vi "rsidr_core_global.vi"() -> ()   [LabVIEW 2020, in "Rohde&Schwarz RTx Oscilloscopes.lvlib"] (continued)
Table"="", "Read Callback"="", "Write Callback"="", "Supported Models"="", "Instrument Options"="K15", "Flags"=0, "Help"="Displays or hides the segment table on the screen.\n\nAvailable Repeated Capabilities:\nMath: MA1, MA2, MA3, MA4, MA5\r\n\nRemote-control command(s):\nCALCulate:MATH<m>:HISTory:TTABle[:ENABle]"}, {"Level"=4, "Class Only"=FALSE, "Identifier"="RSRTX_ATTR_HISTORY_MATH_EXPORT_NAME", "Descriptive Name"="History Math Export Name", "Data Type"=2, "Command"="CALC:MATH{Math}:HIST:EXP:NAME", "Access"=2, "Range Table"="", "Read Callback"="", "Write Callback"="", "Supported Models"="RTM|RTA", "Instrument Options"="", "Flags"=0, "Help"="History export file name.\n\nAvailable Repeated Capabilities:\nMath: MA1, MA2, MA3, MA4, MA5\r\n\nRemote-control command(s):\nCALCulate:MATH<m>:HISTory:EXPort:NAME"}, {"Level"=4, "Class Only"=FALSE, "Identifier"="RSRTX_ATTR_HISTORY_MATH_EXPORT_SAVE", "Descriptive Name"="History Math Export Save", "Data Type"=4, "Command"="CALC:MATH{Math}:HIST:EXP:SAVE", "Access"=1, "Range Table"="", "Read Callback"="", "Write Callback"="", "Supported Models"="RTM|RTA", "Instrument Options"="", "Flags"=0, "Help"="Exports history.\n\nAvailable Repeated Capabilities:\nMath: MA1, MA2, MA3, MA4, MA5\r\n\nRemote-control command(s):\nCALCulate:MATH<m>:HISTory:EXPort:SAVE"}, {"Level"=3, "Class Only"=TRUE, "Identifier"="", "Descriptive Name"="Protocol", "Data Type"=0, "Command"="", "Access"=0, "Range Table"="", "Read Callback"="", "Write Callback"="", "Supported Models"="", "Instrument Options"="", "Flags"=0, "Help"="Configures history for protocol."}, {"Level"=4, "Class Only"=FALSE, "Identifier"="RSRTX_ATTR_HISTORY_PROTOCOL_CURRENT_ACQUISITION", "Descriptive Name"="History Protocol Current Acquisition", "Data Type"=0, "Command"="BUS{SerialBus}:HIST:CURR", "Access"=2, "Range Table"="", "Read Callback"="", "Write Callback"="", "Supported Models"="", "Instrument Options"="K15", "Flags"=0, "Help"="Accesses a particular acquisition segment in the memory to display it. The query returns the index of the segment that is shown.\nThere are two ways to enter the index.\nNegative index count: the newest segment has the index 0, older segments have a negative index: -(n-1), .... -1 , 0\nPositive index count: the oldest segment has the index 1, and the newest segment has the index n: 1, 2,..., n\nwhere n is the number of acquired segments.\n\nAvailable Repeated Capabilities:\nSerialBus: SB1, SB2, SB3, SB4\r\n\nRemote-control command(s):\nBUS<b>:HISTory:CURRent"}, {"Level"=4, "Class Only"=FALSE, "Identifier"="RSRTX_ATTR_HISTORY_PROTOCOL_PLAYER", "Descriptive Name"="History Protocol Player", "Data Type"=0, "Command"="BUS{SerialBus}:HIST:PLAY:STAT", "Access"=2, "Range Table"="rsrtx_rngHistoryPlayer", "Read Callback"="", "Write Callback"="", "Supported Models"="", "Instrument Options"="K15", "Flags"=0, "Help"="Starts and stops the replay of the history segments.\n\nAvailable Repeated Capabilities:\nSerialBus: SB1, SB2, SB3, SB4\r\n\nRemote-control command(s):\nBUS<b>:HISTory:PLAYer:STATe"}, {"Level"=4, "Class Only"=FALSE, "Identifier"="RSRTX_ATTR_HISTORY_PROTOCOL_START_ACQUISITION", "Descriptive Name"="History Protocol Start Acquisition", "Data Type"=0, "Command"="BUS{SerialBus}:HIST:STAR", "Access"=2, "Range Table"="", "Read Callback"="", "Write Callback"="", "Supported Models"="", "Instrument Options"="K15", "Flags"=0, "Help"="Sets the index of the oldest segment to be displayed.\nThere are two ways to enter the index.\nNegative index count: the newest segment has the index 0, older segments have a negative index: -(n-1), .... -1 , 0\nPositive index count: the oldest segment has the index 1, and the newest segment has the index n: 1, 2,..., n\nwhere n is the number of acquired segments.\n\nAvailable Repeated Capabilities:\nSerialBus: SB1, SB2, SB3, SB4\r\n\nRemote-control command(s):\nBUS<b>:HISTory:STARt"}, {"Level"=4, "Class Only"=FALSE, "Identifier"="RSRTX_ATTR_HISTORY_PROTOCOL_STOP_ACQUISITION", "Descriptive Name"="History Protocol Stop Acquisition", "Data Type"=0, "Command"="BUS{SerialBus}:HIST:STOP", "Access"=2, "Range Table"="", "Read Callback"="", "Write Callback"="", "Supported Models"="", "Instrument Options"="K15", "Flags"=0, "Help"="Sets the index of the latest segment to be displayed.\nThere are two ways to enter the index.\nNegative index count: the newest segment has the index 0, older segments have a negative index: -(n-1), .... -1 , 0\nPositive index count: the oldest segment has the index 1, and the newest segment has the index n: 1, 2,..., n\nwhere n is the number of acquired segments.\n\nAvailable Repeated Capabilities:\nSerialBus: SB1, SB2, SB3, SB4\r\n\nRemote-control command(s):\nBUS<b>:HISTory:STOP"}, {"Level"=4, "Class Only"=FALSE, "Identifier"="RSRTX_ATTR_HISTORY_PROTOCOL_PLAY_ALL", "Descriptive Name"="History Protocol Play All", "Data Type"=3, "Command"="BUS{SerialBus}:HIST:PALL", "Access"=2, "Range Table"="", "Read Callback"="", "Write Callback"="", "Supported Models"="", "Instrument Options"="K15", "Flags"=0, "Help"="Enables the replay of all acquired segments.\n\nAvailable Repeated Capabilities:\nSerialBus: SB1, SB2, SB3, SB4\r\n\nRemote-control command(s):\nBUS<b>:HISTory:PALL"}, {"Level"=4, "Class Only"=FALSE, "Identifier"="RSRTX_ATTR_HISTORY_PROTOCOL_SPEED", "Descriptive Name"="History Protocol Speed", "Data Type"=0, "Command"="BUS{SerialBus}:HIST:PLAY:SPE", "Access"=2, "Range Table"="rsrtx_rngHistorySpeed", "Read Callback"="", "Write Callback"="", "Supported Models"="", "Instrument Options"="K15", "Flags"=0, "Help"="Sets the speed of the history replay.\n\nAvailable Repeated Capabilities:\nSerialBus: SB1, SB2, SB3, SB4\r\n\nRemote-control command(s):\nBUS<b>:HISTory:PLAYer:SPEed"}, {"Level"=4, "Class Only"=FALSE, "Identifier"="RSRTX_ATTR_HISTORY_PROTOCOL_REPEAT", "Descriptive Name"="History Protocol Repeat", "Data Type"=3, "Command"="BUS{SerialBus}:HIST:REPL", "Access"=2, "Range Table"="", "Read Callback"="", "Write Callback"="", "Supported Models"="", "Instrument Options"="K15", "Flags"=0, "Help"="If set to true, the replay of the selected history segments repeats automatically.\n\nAvailable Repeated Capabilities:\nSerialBus: SB1, SB2, SB3, SB4\r\n\nRemote-control command(s):\nBUS<b>:HISTory:REPLay"}, {"Level"=4, "Class Only"=FALSE, "Identifier"="RSRTX_ATTR_HISTORY_PROTOCOL_ACQUISITON_RELATIVE_TIME", "Descriptive Name"="History Protocol Acquisiton Relative Time", "Data Type"=1, "Command"="BUS{SerialBus}:HIST:TSR?", "Access"=0, "Range Table"="", "Read Callback"="", "Write Callback"="", "Supported Models"="", "Instrument Options"="K15", "Flags"=0, "Help"="Returns the time difference of the selected segment to the newest segment.\n\nAvailable Repeated Capabilities:\nSerialBus: SB1, SB2, SB3, SB4\r\n\nRemote-control command(s):\nBUS<b>:HISTory:TSRelative?"}, {"Level"=4, "Class Only"=FALSE, "Identifier"="RSRTX_ATTR_HISTORY_PROTOCOL_ALL_DATES", "Descriptive Name"="History Protocol All Dates", "Data Type"=2, "Command"="BUS{SerialBus}:HIST:TSD:ALL?", "Access"=0, "Range Table"="", "Read Callback"="", "Write Callback"="", "Supported Models"="", "Instrument Options"="", "Flags"=0, "Help"="Returns the dates of all history segments.\n\nAvailable Repeated Capabilities:\nSerialBus: SB1, SB2, SB3, SB4\r\n\nRemote-control command(s):\nBUS<b>:HISTory:TSDate:ALL?"}, {"Level"=4, "Class Only"=FALSE, "Identifier"="RSRTX_ATTR_HISTORY_PROTOCOL_ALL_TIME_DIFFERENCES", "Descriptive Name"="History Protocol All Time Differences", "Data Type"=2, "Command"="BUS{SerialBus}:HIST:TSR:ALL?", "Access"=0, "Range Table"="", "Read Callback"="", "Write Callback"="", "Supported Models"="", "Instrument Options"="", "Flags"=0, "Help"="Returns the time differences to the newest acquisition of all history segments.\n\nAvailable Repeated Capabilities:\nSerialBus: SB1, SB2, SB3, SB4\r\n\nRemote-control command(s):\nBUS<b>:HISTory:TSRelative:ALL?"}, {"Level"=4, "Class Only"=FALSE, "Identifier"="RSRTX_ATTR_HISTORY_PROTOCOL_ALL_DAYTIMES", "Descriptive Name"="History Protocol All Daytimes", "Data Type"=2, "Command"="BUS{SerialBus}:HIST:TSAB:ALL?", "Access"=0, "Range Table"="", "Read Callback"="", "Write Callback"="", "Supported Models"="", "Instrument Options"="", "Flags"=0, "Help"="Returns the absolute daytimes of all history segments.\n\nAvailable Repeated Capabilities:\nSerialBus: SB1, SB2, SB3, SB4\r\n\nRemote-control command(s):\nBUS<b>:HISTory:TSABsolute:ALL?"}, {"Level"=4, "Class Only"=FALSE, "Identifier"="RSRTX_ATTR_HISTORY_PROTOCOL_PLAYER_CONTROL_ENABLE", "Descriptive Name"="History Protocol Player Control Enable", "Data Type"=3, "Command"="BUS{SerialBus}:HIST:CONT", "Access"=2, "Range Table"="", "Read Callback"="", "Write Callback"="", "Supported Models"="", "Instrument Options"="K15", "Flags"=0, "Help"="Displays or hides the history player on the screen.\n\nAvailable Repeated Capabilities:\nSerialBus: SB1, SB2, SB3, SB4\r\n\nRemote-control command(s):\nBUS<b>:HISTory:CONTrol[:ENABle]"}, {"Level"=4, "Class Only"=FALSE, "Identifier"="RSRTX_ATTR_HISTORY_PROTOCOL_TIME_TABLE_ENABLE", "Descriptive Name"="History Protocol Time Table Enable", "Data Type"=3, "Command"="BUS{SerialBus}:HIST:TTAB", "Access"=2, "Range Table"="", "Read Callback"="", "Write Callback"="", "Supported Models"="", "Instrument Options"="K15", "Flags"=0, "Help"="Displays or hides the segment table on the screen.\n\nAvailable Repeated Capabilities:\nSerialBus: SB1, SB2, SB3, SB4\r\n\nRemote-control command(s):\nBUS<b>:HISTory:TTABle[:ENABle]"}, {"Level"=4, "Class Only"=FALSE, "Identifier"="RSRTX_ATTR_HISTORY_PROTOCOL_EXPORT_NAME", "Descriptive Name"="History Protocol Export Name", "Data Type"=2, "Command"="BUS{SerialBus}:HIST:EXP:NAME", "Access"=2, "Range Table"="", "Read Callback"="", "Write Callback"="", "Supported Models"="", "Instrument Options"="", "Flags"=0, "Help"="History export file name.\n\nAvailable Repeated Capabilities:\nSerialBus: SB1, SB2, SB3, SB4\r\n\nRemote-control command(s):\nBUS<b>:HISTory:EXPort:NAME"}, {"Level"=4, "Class Only"=FALSE, "Identifier"="RSRTX_ATTR_HISTORY_PROTOCOL_EXPORT_SAVE", "Descriptive Name"="History Protocol Export Save", "Data Type"=4, "Command"="BUS{SerialBus}:HIST:EXP:SAVE", "Access"=1, "Range Table"="", "Read Callback"="", "Write Callback"="", "Supported Models"="", "Instrument Options"="", "Flags"=0, "Help"="Exports history.\n\nAvailable Repeated Capabilities:\nSerialBus: SB1, SB2, SB3, SB4\r\n\nRemote-control command(s):\nBUS<b>:HISTory:EXPort:SAVE"}, {"Level"=3, "Class Only"=TRUE, "Identifier"="", "Descriptive Name"="Spectrum", "Data Type"=0, "Command"="", "Access"=0, "Range Table"="", "Read Callback"="", "Write Callback"="", "Supported Models"="", "Instrument Options"="", "Flags"=0, "Help"="Contains attributes for Spectrum History."}, {"Level"=4, "Class Only"=FALSE, "Identifier"="RSRTX_ATTR_HISTORY_SPECTRUM_CURRENT_ACQUISITION", "Descriptive Name"="History Spectrum Current Acquisition", "Data Type"=0, "Command"="SPEC:HIST:CURR", "Access"=2, "Range Table"="", "Read Callback"="", "Write Callback"="", "Supported Models"="", "Instrument Options"="K15", "Flags"=0, "Help"="Accesses a particular acquisition segment in the memory to display it. The query returns the index of the segment that is shown.\n\nAvailable Repeated Capabilities:\nNone\n\nRemote-control command(s):\nSPECtrum:HISTory:CURRent"}, {"Level"=4, "Class Only"=FALSE, "Identifier"="RSRTX_ATTR_HISTORY_SPECTRUM_PLAYER", "Descriptive Name"="History Spectrum Player", "Data Type"=0, "Command"="SPEC:HIST:PLAY:STAT", "Access"=2, "Range Table"="rsrtx_rngHistoryPlayer", "Read Callback"="", "Write Callback"="", "Supported Models"="", "Instrument Options"="K15", "Flags"=0, "Help"="Starts and stops the replay of the history segments.\n\nAvailable Repeated Capabilities:\nNone\n\nRemote-control command(s):\nSPECtrum:HISTory:PLAYer:STATe"}, {"Level"=4, "Class Only"=FALSE, "Identifier"="RSRTX_ATTR_HISTORY_SPECTRUM_START_ACQUISITION", "Descriptive Name"="History Spectrum Start Acquisition", "Data Type"=0, "Command"="SPEC:HIST:STAR", "Access"=2, "Range Table"="", "Read Callback"="", "Write Callback"="", "Supported Models"="", "Instrument Options"="K15", "Flags"=0, "Help"="Sets the index of the oldest segment to be displayed.\nThere are two ways to enter the index.\nNegative index count: the newest segment has the index 0, older segments have a negative index: -(n-1), .... -1 , 0\nPositive index count: the oldest segment has the index 1, and the newest segment has the index n: 1, 2,..., n\nwhere n is the number of acquired segments.\n\nAvailable Repeated Capabilities:\nNone\n\nRemote-control command(s):\nSPECtrum:HISTory:STARt"}, {"Level"=4, "Class Only"=FALSE, "Identifier"="RSRTX_ATTR_HISTORY_SPECTRUM_STOP_ACQUISITION", "Descriptive Name"="History Spectrum Stop Acquisition", "Data Type"=0, "Command"="SPEC:HIST:STOP", "Access"=2, "Range Table"="", "Read Callback"="", "Write Callback"="", "Supported Models"="", "Instrument Options"="K15", "Flags"=0, "Help"="Sets the index of the latest segment to be displayed.\nThere are two ways to enter the index.\nNegative index count: the newest segment has the index 0, older segments have a negative index: -(n-1), .... -1 , 0\nPositive index count: the oldest segment has the index 1, and the newest segment has the index n: 1, 2,..., n\nwhere n is the number of acquired segments.\n\nAvailable Repeated Capabilities:\nNone\n\nRemote-control command(s):\nSPECtrum:HISTory:STOP"}, {"Level"=4, "Class Only"=FALSE, "Identifier"="RSRTX_ATTR_HISTORY_SPECTRUM_PLAY_ALL", "Descriptive Name"="History Spectrum Play All", "Data Type"=3, "Command"="SPEC:HIST:PALL", "Access"=2, "Range Table"="", "Read Callback"="", "Write Callback"="", "Supported Models"="", "Instrument Options"="K15", "Flags"=0, "Help"="Enables the replay of all acquired segments.\n\nAvailable Repeated Capabilities:\nNone\n\nRemote-control command(s):\nSPECtrum:HISTory:PALL"}, {"Level"=4, "Class Only"=FALSE, "Identifier"="RSRTX_ATTR_HISTORY_SPECTRUM_SPEED", "Descriptive Name"="History Spectrum Speed", "Data Type"=0, "Command"="SPEC:HIST:PLAY:SPE", "Access"=2, "Range Table"="rsrtx_rngHistorySpeed", "Read Callback"="", "Write Callback"="", "Supported Models"="", "Instrument Options"="K15", "Flags"=0, "Help"="Sets the speed of the history replay.\n\nAvailable Repeated Capabilities:\nNone\n\nRemote-control command(s):\nSPECtrum:HISTory:PLAYer:SPEed"}, {"Level"=4, "Class Only"=FALSE, "Identifier"="RSRTX_ATTR_HISTORY_SPECTRUM_REPEAT", "Descriptive Name"="History Spectrum Repeat", "Data Type"=3, "Command"="SPEC:HIST:REPL", "Access"=2, "Range Table"="", "Read Callback"="", "Write Callback"="", "Supported Models"="", "Instrument Options"="K15", "Flags"=0, "Help"="If set to true, the replay of the selected history segments repeats automatically.\n\nAvailable Repeated Capabilities:\nNone\n\nRemote-control command(s):\nSPECtrum:HISTory:REPLay"}, {"Level"=4, "Class Only"=FALSE, "Identifier"="RSRTX_ATTR_HISTORY_SPECTRUM_ACQUISITION_RELATIVE_TIME", "Descriptive Name"="History Spectrum Acquisition Relative Time", "Data Type"=1, "Command"="SPEC:HIST:TSR?", "Access"=0, "Range Table"="", "Read Callback"="", "Write Callback"="", "Supported Models"="", "Instrument Options"="", "Flags"=0, "Help"="Returns the time difference of the selected segment to the newest segment. To select a segment, use RSRTX_ATTR_HISTORY_CHANNEL_CURRENT_ACQUISITION. The newest segment has index 0.\n\nAvailable Repeated Capabilities:\nNone\n\nRemote-control command(s):\nSPECtrum:HISTory:TSRelative?"}, {"Level"=4, "Class Only"=FALSE, "Identifier"="RSRTX_ATTR_HISTORY_SPECTRUM_ALL_DATES", "Descriptive Name"="History Spectrum All Dates", "Data Type"=2, "Command"="SPEC:HIST:TSD:ALL?", "Access"=0, "Range Table"="", "Read Callback"="", "Write Callback"="", "Supported Models"="", "Instrument Options"="", "Flags"=0, "Help"="Returns the dates of all history segments as a list of comma-separated list of year, month, and day values. The list starts with the oldest segment, and the newest segment is the last one.\n\nAvailable Repeated Capabilities:\nNone\n\nRemote-control command(s):\nSPECtrum:HISTory:TSDate:ALL?"}, {"Level"=4, "Class Only"=FALSE, "Identifier"="RSRTX_ATTR_HISTORY_SPECTRUM_ALL_TIME_DIFFERENCES", "Descriptive Name"="History Spectrum All Time Differences", "Data Type"=2, "Command"="SPEC:HIST:TSR:ALL?", "Access"=0, "Range Table"="", "Read Callback"="", "Write Callback"="", "Supported Models"="", "Instrument Options"="", "Flags"=0, "Help"="Returns the time differences to the newest acquisition of all history segments.\n\nAvailable Repeated Capabilities:\nNone\n\nRemote-control command(s):\nSPECtrum:HISTory:TSRelative:ALL?"}, {"Level"=4, "Class Only"=FALSE, "Identifier"="RSRTX_ATTR_HISTORY_SPECTRUM_ALL_DAYTIMES", "Descriptive Name"="History Spectrum All Daytimes", "Data Type"=2, "Command"="SPEC:HIST:TSAB:ALL?", "Access"=0, "Range Table"="", "Read Callback"="", "Write Callback"="", "Supported Models"="", "Instrument Options"="", "Flags"=0, "Help"="Returns the absolute daytimes of all history segments.\n\nAvailable Repeated Capabilities:\nNone\n\nRemote-control command(s):\nSPECtrum:HISTory:TSABsolute:ALL?"}, {"Level"=4, "Class Only"=FALSE, "Identifier"="RSRTX_ATTR_HISTORY_SPECTRUM_EXPORT_NAME", "Descriptive Name"="History Spectrum Export Name", "Data Type"=2, "Command"="SPEC:HIST:EXP:NAME", "Access"=2, "Range Table"="", "Read Callback"="", "Write Callback"="", "Supported Models"="", "Instrument Options"="K15", "Flags"=0, "Help"="Defines the path and filename of the spectrum analysis timestamps file. The file format is CSV. If the file already exists, it will be overwritten.\n\nAvailable Repeated Capabilities:\nNone\n\nRemote-control command(s):\nSPECtrum:HISTory:EXPort:NAME"}, {"Level"=4, "Class Only"=FALSE, "Identifier"="RSRTX_ATTR_HISTORY_SPECTRUM_EXPORT_SAVE", "Descriptive Name"="History Spectrum Export Save", "Data Type"=4, "Command"="SPEC:HIST:EXP:SAVE", "Access"=1, "Range Table"="", "Read Callback"="", "Write Callback"="", "Supported Models"="", "Instrument Options"="K15", "Flags"=0, "Help"="Saves the spectrum analysis timestamps table to the file that is defined by the SPECtrum:HISTory:EXPort:NAME command.\n\nAvailable Repeated Capabilities:\nNone\n\nRemote-control command(s):\nSPECtrum:HISTory:EXPort:SAVE"}, {"Level"=3, "Class Only"=TRUE, "Identifier"="", "Descriptive Name"="Logic", "Data Type"=0, "Command"="", "Access"=0, "Range Table"="", "Read Callback"="", "Write Callback"="", "Supported Models"="", "Instrument Options"="", "Flags"=0, "Help"="Configures history for logic probe."}, {"Level"=4, "Class Only"=FALSE, "Identifier"="RSRTX_ATTR_HISTORY_LOGIC_CURRENT_ACQUISITION", "Descriptive Name"="History Logic Current Acquisition", "Data Type"=0, "Command"="LOG{Logic}:HIST:CURR", "Access"=2, "Range Table"="", "Read Callback"="", "Write Callback"="", "Supported Models"="", "Instrument Options"="K15", "Flags"=0, "Help"="Accesses a particular acquisition segment in the memory to display it. The query returns the index of the segment that is shown.\nThere are two ways to enter the index.\nNegative index count: the newest segment has the index 0, older segments have a negative index: -(n-1), .... -1 , 0\nPositive index count: the oldest segment has the index 1, and the newest segment has the index n: 1, 2,..., n\nwhere n is the number of acquired segments.\n\nAvailable Repeated Capabilities:\nLogic: Logic1, Logic2\r\n\nRemote-control command(s):\nLOGic<p>:HISTory:CURRent"}, {"Level"=4, "Class Only"=FALSE, "Identifier"="RSRTX_ATTR_HISTORY_LOGIC_PLAYER", "Descriptive Name"="History Logic Player", "Data Type"=0, "Command"="LOG{Logic}:HIST:PLAY:STAT", "Access"=2, "Range Table"="rsrtx_rngHistoryPlayer", "Read Callback"="", "Write Callback"="", "Supported Models"="", "Instrument Options"="K15", "Flags"=0, "Help"="Starts and stops the replay of the history segments.\n\nAvailable Repeated Capabilities:\nLogic: Logic1, Logic2\r\n\nRemote-control command(s):\nLOGic<p>:HISTory:PLAYer:STATe"}, {"Level"=4, "Class Only"=FALSE, "Identifier"="RSRTX_ATTR_HISTORY_LOGIC_START_ACQUISITION", "Descriptive Name"="History Logic Start Acquisition", "Data Type"=0, "Command"="LOG{Logic}:HIST:STAR", "Access"=2, "Range Table"="", "Read Callback"="", "Write Callback"="", "Supported Models"="", "Instrument Options"="K15", "Flags"=0, "Help"="Sets the index of the oldest segment to be displayed.\nThere are two ways to enter the index.\nNegative index count: the newest segment has the index 0, older segments have a negative index: -(n-1), .... -1 , 0\nPositive index count: the oldest segment has the index 1, and the newest segment has the index n: 1, 2,..., n\nwhere n is the number of acquired segments.\n\nAvailable Repeated Capabilities:\nLogic: Logic1, Logic2\r\n\nRemote-control command(s):\nLOGic<p>:HISTory:STARt"}, {"Level"=4, "Class Only"=FALSE, "Identifier"="RSRTX_ATTR_HISTORY_LOGIC_STOP_ACQUISITION", "Descriptive Name"="History Logic Stop Acquisition", "Data Type"=0, "Command"="LOG{Logic}:HIST:STOP", "Access"=2, "Range Table"="", "Read Callback"="", "Write Callback"="", "Supported Models"="", "Instrument Options"="K15", "Flags"=0, "Help"="Sets the index of the latest segment to be displayed.\nThere are two ways to enter the index.\nNegative index count: the newest segment has the index 0, older segments have a negative index: -(n-1), .... -1 , 0\nPositive index count: the oldest segment has the index 1, and the newest segment has the index n: 1, 2,..., n\nwhere n is the number of acquired segments.\n\nAvailable Repeated Capabilities:\nLogic: Logic1, Logic2\r\n\nRemote-control command(s):\nLOGic<p>:HISTory:STOP"}, {"Level"=4, "Class Only"=FALSE, "Identifier"="RSRTX_ATTR_HISTORY_LOGIC_PLAY_ALL", "Descriptive Name"="History Logic Play All", "Data Type"=3, "Command"="LOG{Logic}:HIST:PALL", "Access"=2, "Range Table"="", "Read Callback"="", "Write Callback"="", "Supported Models"="", "Instrument Options"="K15", "Flags"=0, "Help"="Enables the replay of all acquired segments.\n\nAvailable Repeated Capabilities:\nLogic: Logic1, Logic2\r\n\nRemote-control command(s):\nLOGic<p>:HISTory:PALL"}, {"Level"=4, "Class Only"=FALSE, "Identifier"="RSRTX_ATTR_HISTORY_LOGIC_SPEED", "Descriptive Name"="History Logic Speed", "Data Type"=0, "Command"="LOG{Logic}:HIST:PLAY:SPE", "Access"=2, "Range Table"="rsrtx_rngHistorySpeed", "Read Callback"="", "Write Callback"="", "Supported Models"="", "Instrument Options"="K15", "Flags"=0, "Help"="Sets the speed of the history replay.\n\nAvailable Repeated Capabilities:\nLogic: Logic1, Logic2\r\n\nRemote-control command(s):\nLOGic<p>:HISTory:PLAYer:SPEed"}, {"Level"=4, "Class Only"=FALSE, "Identifier"="RSRTX_ATTR_HISTORY_LOGIC_REPEAT", "Descriptive Name"="History Logic Repeat", "Data Type"=3, "Command"="LOG{Logic}:HIST:REPL", "Access"=2, "Range Table"="", "Read Callback"="", "Write Callback"="", "Supported Models"="", "Instrument Options"="K15", "Flags"=0, "Help"="If set to true, the replay of the selected history segments repeats automatically.\n\nAvailable Repeated Capabilities:\nLogic: Logic1, Logic2\r\n\nRemote-control command(s):\nLOGic<p>:HISTory:REPLay"}, {"Level"=4, "Class Only"=FALSE, "Identifier"="RSRTX_ATTR_HISTORY_LOGIC_ACQUISITON_RELATIVE_TIME", "Descriptive Name"="History Logic Acquisiton Relative Time", "Data Type"=1, "Command"="LOG{Logic}:HIST:TSR?", "Access"=0, "Range Table"="", "Read Callback"="", "Write Callback"="", "Supported Models"="", "Instrument Options"="K15", "Flags"=0, "Help"="Returns the time difference of the selected segment to the newest segment.\n\nAvailable Repeated Capabilities:\nLogic: Logic1, Logic2\r\n\nRemote-control command(s):\nLOGic<p>:HISTory:TSRelative?"}, {"Level"=4, "Class Only"=FALSE, "Identifier"="RSRTX_ATTR_HISTORY_LOGIC_ALL_DATES", "Descriptive Name"="History Logic All Dates", "Data Type"=2, "Command"="LOG{Logic}:HIST:TSR:ALL?", "Access"=0, "Range Table"="", "Read Callback"="", "Write Callback"="", "Supported Models"="", "Instrument Options"="", "Flags"=0, "Help"="Returns the dates of all history segments.\n\nAvailable Repeated Capabilities:\nLogic: Logic1, Logic2\r\n\nRemote-control command(s):\nLOGic<p>:HISTory:TSRelative:ALL?"}, {"Level"=4, "Class Only"=FALSE, "Identifier"="RSRTX_ATTR_HISTORY_LOGIC_ALL_TIME_DIFFERENCES", "Descriptive Name"="History Logic All Time Differences", "Data Type"=2, "Command"="LOG{Logic}:HIST:TSD:ALL?", "Access"=0, "Range Table"="", "Read Callback"="", "Write Callback"="", "Supported Models"="", "Instrument Options"="K15", "Flags"=0, "Help"="Returns the time differences to the newest acquisition of all history segments.\n\nAvailable Repeated Capabilities:\nLogic: Logic1, Logic2\r\n\nRemote-control command(s):\nLOGic<p>:HISTory:TSDate:ALL?"}, {"Level"=4, "Class Only"=FALSE, "Identifier"="RSRTX_ATTR_HISTORY_LOGIC_ALL_DAYTIMES", "Descriptive Name"="History Logic All Daytimes", "Data Type"=2, "Command"="LOG{Logic}:HIST:TSAB:ALL?", "Access"=0, "Range Table"="", "Read Callback"="", "Write Callback"="", "Supported Models"="", "Instrument Options"="", "Flags"=0, "Help"="Returns the absolute daytimes of all history segments.\n\nAvailable Repeated Capabilities:\nLogic: Logic1, Logic2\r\n\nRemote-control command(s):\nLOGic<p>:HISTory:TSABsolute:ALL?"}, {"Level"=4, "Class Only"=FALSE, "Identifier"="RSRTX_ATTR_HISTORY_LOGIC_PLAYER_CONTROL_ENABLE", "Descriptive Name"="History Logic Player Control Enable", "Data Type"=3, "Command"="LOG{Logic}:HIST:CONT", "Access"=2, "Range Table"="", "Read Callback"="", "Write Callback"="", "Supported Models"="", "Instrument Options"="K15", "Flags"=0, "Help"="Displays or hides the history player on the screen.\n\nAvailable Repeated Capabilities:\nLogic: Logic1, Logic2\r\n\nRemote-control command(s):\nLOGic<p>:HISTory:CONTrol[:ENABle]"}, {"Level"=4, "Class Only"=FALSE, "Identifier"="RSRTX_ATTR_HISTORY_LOGIC_TIME_TABLE_ENABLE", "Descriptive Name"="History Logic Time Table Enable", "Data Type"=3, "Command"="LOG{Logic}:HIST:TTAB", "Access"=2, "Range Table"="", "Read Callback"="", "Write Callback"="", "Supported Models"="", "Instrument Options"="K15", "Flags"=0, "Help"="Displays or hides the segment table on the screen.\n\nAvailable Repeated Capabilities:\nLogic: Logic1, Logic2\r\n\nRemote-control command(s):\nLOGic<p>:HISTory:TTABle[:ENABle]"}, {"Level"=4, "Class Only"=FALSE, "Identifier"="RSRTX_ATTR_HISTORY_LOGIC_EXPORT_NAME", "Descriptive Name"="History Logic Export Name", "Data Type"=2, "Command"="LOG{Logic}:HIST:EXP:NAME", "Access"=2, "Range Table"="", "Read Callback"="", "Write Callback"="", "Supported Models"="", "Instrument Options"="K15", "Flags"=0, "Help"="History export file name.\n\nAvailable Repeated Capabilities:\nLogic: Logic1, Logic2\r\n\nRemote-control command(s):\nLOGic<p>:HISTory:EXPort:NAME"}, {"Level"=4, "Class Only"=FALSE, "Identifier"="RSRTX_ATTR_HISTORY_LOGIC_EXPORT_SAVE", "Descriptive Name"="History Logic Export Save", "Data Type"=4, "Command"="LOG{Logic}:HIST:EXP:SAVE", "Access"=1, "Range Table"="", "Read Callback"="", "Write Callback"="", "Supported Models"="", "Instrument Options"="K15", "Flags"=0, "Help"="Exports history.\n\nAvailable Repeated Capabilities:\nLogic: Logic1, Logic2\r\n\nRemote-control command(s):\nLOGic<p>:HISTory:EXPort:SAVE"}, {"Level"=2, "Class Only"=TRUE, "Identifier"="", "Descriptive Name"="Segmentation", "Data Type"=0, "Command"="", "Access"=0, "Range Table"="", "Read Callback"="", "Write Callback"="", "Supported Models"="", "Instrument Options"="", "Flags"=0, "Help"="Configures Display Segmentation."}, {"Level"=3, "Class Only"=FALSE, "Identifier"="RSRTX_ATTR_SEGMENTATION_RECORD_LENGTH", "Descriptive Name"="Segmentation Record Length", "Data Type"=0, "Command"="ACQ:POIN", "Access"=2, "Range Table"="", "Read Callback"="", "Write Callback"="", "Supported Models"="", "Instrument Options"="K15", "Flags"=0, "Help"="Record length, the number of recorded waveform points in a segment.\n\nAvailable Repeated Capabilities:\nNone\n\nRemote-control command(s):\nACQuire:POINts[:VALue]"}, {"Level"=3, "Class Only"=FALSE, "Identifier"="RSRTX_ATTR_ULTRA_SEGMENTATION_ENABLED", "Descriptive Name"="Ultra Segmentation Enabled", "Data Type"=3, "Command"="ACQ:SEGM:STAT", "Access"=2, "Range Table"="", "Read Callback"="", "Write Callback"="", "Supported Models"="", "Instrument Options"="K15", "Flags"=0, "Help"="Enables the ultra segementation mode. The acquisitions are performed very fast without processing and displaying the waveforms. When acquisition has been stopped, the latest waveform is displayed, the older ones are stored in segments.\n\nAvailable Repeated Capabilities:\nNone\n\nRemote-control command(s):\nACQuire:SEGMented:STATe"}, {"Level"=3, "Class Only"=FALSE, "Identifier"="RSRTX_ATTR_SEGMENTATION_RECORD_MAXIMUM_SEGMENTS", "Descriptive Name"="Segmentation Record Maximum Segments", "Data Type"=3, "Command"="ACQ:SEGM:MAX", "Access"=2, "Range Table"="", "Read Callback"="", "Write Callback"="", "Supported Models"="", "Instrument Options"="", "Flags"=0, "Help"="Always records maximum possible number of segments.\n\nAvailable Repeated Capabilities:\nNone\n\nRemote-control command(s):\nACQuire:SEGMented:MAXimum"}, {"Level"=3, "Class Only"=FALSE, "Identifier"="RSRTX_ATTR_SEGMENTATION_NX_SINGLE_MAXIMUM", "Descriptive Name"="Segmentation Nx Single Maximum", "Data Type"=3, "Command"="ACQ:NSIN:MAX", "Access"=2, "Range Table"="", "Read Callback"="", "Write Callback"="", "Supported Models"="", "Instrument Options"="K15", "Flags"=0, "Help"="Sets the maximum possible number of segments for a RUN Nx SINGLE acquisition.\nThus, all segments of the memory are captured.\n\nAvailable Repeated Capabilities:\nNone\n\nRemote-control command(s):\nACQuire:NSINgle:MAXimum"}, {"Level"=3, "Class Only"=FALSE, "Identifier"="RSRTX_ATTR_SEGMENTATION_MAXIMUM_NUMBER_OF_SEGMENTS", "Descriptive Name"="Segmentation Maximum Number Of Segments", "Data Type"=0, "Command"="ACQ:COUN", "Access"=2, "Range Table"="", "Read Callback"="", "Write Callback"="", "Supported Models"="", "Instrument Options"="K15", "Flags"=0, "Help"="Sets the number of segments to be captured. In automatic mode, the command is query only and returns the maximum number of segments that can be captured with the current configuration.\n\nAvailable Repeated Capabilities:\nNone\n\nRemote-control command(s):\nACQuire:COUNt"}, {"Level"=3, "Class Only"=FALSE, "Identifier"="RSRTX_ATTR_SEGMENTATION_NUMBER_OF_AVAILABLE_SEGMENTS", "Descriptive Name"="Segmentation Number Of Available Segments", "Data Type"=0, "Command"="ACQ:AVA?", "Access"=0, "Range Table"="", "Read Callback"="", "Write Callback"="", "Supported Models"="", "Instrument Options"="K15", "Flags"=0, "Help"="Returns the number of segments that are currently saved in the memory. This number is available for history viewing.\n\nAvailable Repeated Capabilities:\nNone\n\nRemote-control command(s):\nACQuire:AVAilable?"}, {"Level"=1, "Class Only"=TRUE, "Identifier"="", "Descriptive Name"="Data Management", "Data Type"=0, "Command"="", "Access"=0, "Range Table"="", "Read Callback"="", "Write Callback"="", "Supported Models"="", "Instrument Options"="", "Flags"=0, "Help"="Mass memory, save and load"}, {"Level"=2, "Class Only"=FALSE, "Identifier"="RSRTX_ATTR_DRIVES", "Descriptive Name"="Drives", "Data Type"=2, "Command"="MMEM:DRIV?", "Access"=0, "Range Table"="", "Read Callback"="", "Write Callback"="", "Supported Models"="", "Instrument Options"="", "Flags"=0, "Help"="Returns a list of the drives of the instrument.\n\nAvailable Repeated Capabilities:\nNone\n\nRemote-control command(s):\nMMEMory:DRIVes?"}, {"Level"=2, "Class Only"=FALSE, "Identifier"="RSRTX_ATTR_CHANGE_DRIVE", "Descriptive Name"="Change Drive", "Data Type"=2, "Command"="MMEM:MSIS", "Access"=1, "Range Table"="", "Read Callback"="", "Write Callback"="", "Supported Models"="", "Instrument Options"="", "Flags"=1, "Help"="Change current drive.\n\nAvailable Repeated Capabilities:\nNone\n\nRemote-control command(s):\nMMEMory:MSIS"}, {"Level"=2, "Class Only"=FALSE, "Identifier"="RSRTX_ATTR_CURRENT_DIRECTORY", "Descriptive Name"="Current Directory", "Data Type"=2, "Command"="MMEM:CDIR", "Access"=2, "Range Table"="", "Read Callback"="", "Write Callback"="", "Supported Models"="", "Instrument Options"="", "Flags"=1, "Help"="Changes the default directory for mass memory storage.\n\nAvailable Repeated Capabilities:\nNone\n\nRemote-control command(s):\nMMEMory:CDIRectory"}, {"Level"=2, "Class Only"=FALSE, "Identifier"="RSRTX_ATTR_CREATE_DIRECTORY", "Descriptive Name"="Create Directory", "Data Type"=2, "Command"="MMEM:MDIR", "Access"=1, "Range Table"="", "Read Callback"="", "Write Callback"="", "Supported Models"="", "Instrument Options"="", "Flags"=1, "Help"="Creates a new directory for mass memory storage.\n\nAvailable Repeated Capabilities:\nNone\n\nRemote-control command(s):\nMMEMory:MDIRectory"}, {"Level"=2, "Class Only"=FALSE, "Identifier"="RSRTX_ATTR_REMOVE_DIRECTORY", "Descriptive Name"="Remove Directory", "Data Type"=2, "Command"="MMEM:RDIR", "Access"=1, "Range Table"="", "Read Callback"="", "Write Callback"="", "Supported Models"="", "Instrument Options"="", "Flags"=1, "Help"="Removes an existing directory from the mass memory storage system.\n\nAvailable Repeated Capabilities:\nNone\n\nRemote-control command(s):\nMMEMory:RDIRectory"}, {"Level"=2, "Class Only"=FALSE, "Identifier"="RSRTX_ATTR_DELETE_FILE", "Descriptive Name"="Delete File", "Data Type"=2, "Command"="MMEM:DEL", "Access"=1, "Range Table"="", "Read Callback"="", "Write Callback"="", "Supported Models"="", "Instrument Options"="", "Flags"=1, "Help"="Removes a file from the specified directory.\n\nAvailable Repeated Capabilities:\nNone\n\nRemote-control command(s):\nMMEMory:DELete"}, {"Level"=1, "Class Only"=TRUE, "Identifier"="", "Descriptive Name"="Hardcopy and Printer", "Data Type"=0, "Command"="", "Access"=0, "Range Table"="", "Read Callback"="", "Write Callback"="", "Supported Models"="", "Instrument Options"="", "Flags"=0, "Help"="Contains attributes for Hardcopy and printers setup."}, {"Level"=2, "Class Only"=FALSE, "Identifier"="RSRTX_ATTR_HARDCOPY_FILE_NAME", "Descriptive Name"="Hardcopy File Name", "Data Type"=2, "Command"="MMEM:NAME", "Access"=2, "Range Table"="", "Read Callback"="", "Write Callback"="", "Supported Models"="", "Instrument Options"="", "Flags"=0, "Help"="Defines the file name when an image of the display is stored to a file rather than printed to a printer using RSRTX_ATTR_HARDCOPY_PRINT.\n\nAvailable Repeated Capabilities:\nNone\n\nRemote-control command(s):\nMMEMory:NAME"}, {"Level"=2, "Class Only"=FALSE, "Identifier"="RSRTX_ATTR_HARDCOPY_DEVICE_DESTINATION", "Descriptive Name"="Hardcopy Device Destination", "Data Type"=0, "Command"="HCOP:DEST", "Access"=2, "Range Table"="rsrtx_rngHardcopyDevice", "Read Callback"="", "Write Callback"="", "Supported Models"="", "Instrument Options"="", "Flags"=0, "Help"="Selects the printer output medium (Disk, Printer or Clipboard).\n\nThe type of instrument is selected with SYSTem:COMMunicate:PRINter:SELect<1..2>, which automatically selects a default output medium. Therefore the HCOPy:DESTination command should always be sent after setting the device type.\n\nAvailable Repeated Capabilities:\nNone\n\nRemote-control command(s):\nHCOPy:DESTination"}, {"Level"=2, "Class Only"=FALSE, "Identifier"="RSRTX_ATTR_SCREENSHOT_EXPORT_DESTINATION", "Descriptive Name"="Screenshot Export Destination", "Data Type"=2, "Command"="EXP:SCRS:DEST", "Access"=2, "Range Table"="", "Read Callback"="", "Write Callback"="", "Supported Models"="", "Instrument Options"="", "Flags"=0, "Help"="Defines the directory where screenshots are saved. The specified directory must exist before the command is sent.\n\nAvailable Repeated Capabilities:\nNone\n\nRemote-control command(s):\nEXPort:SCRSave:DESTination"}, {"Level"=2, "Class Only"=FALSE, "Identifier"="RSRTX_ATTR_HARDCOPY_COLOR_SCHEME", "Descriptive Name"="Hardcopy Color Scheme", "Data Type"=0, "Command"="HCOP:COL:SCH", "Access"=2, "Range Table"="rsrtx_rngColorScheme", "Read Callback"="", "Write Callback"="", "Supported Models"="", "Instrument Options"="", "Flags"=0, "Help"="Defines the color mode for saved and printed screenshots.\n\nAvailable Repeated Capabilities:\nNone\n\nRemote-control command(s):\nHCOPy:COLor:SCHeme"}, {"Level"=2, "Class Only"=FALSE, "Identifier"="RSRTX_ATTR_HARDCOPY_COMMAND_SET", "Descriptive Name"="Hardcopy Command Set", "Data Type"=0, "Command"="SYST:COMM:PRIN:CSET", "Access"=2, "Range Table"="rsrtx_rngHardcopyCommandSet", "Read Callback"="", "Write Callback"="", "Supported Models"="", "Instrument Options"="", "Flags"=0, "Help"="Sets the printer language that is supported by the printer.\n\nAvailable Repeated Capabilities:\nNone\n\nRemote-control command(s):\nSYSTem:COMMunicate:PRINter:CSET"}, {"Level"=2, "Class Only"=FALSE, "Identifier"="RSRTX_ATTR_HARDCOPY_CLOSE_DIALOGS", "Descriptive Name"="Hardcopy Close Dialogs", "Data Type"=3, "Command"="HCOP:CWIN", "Access"=2, "Range Table"="", "Read Callback"="", "Write Callback"="", "Supported Models"="", "Instrument Options"="", "Flags"=0, "Help"="If ON, open dialog boxes and menus are closed before the screenshot is saved. Thus, the waveforms and results are always visible on the screenshot.\n\nAvailable Repeated Capabilities:\nNone\n\nRemote-control command(s):\nHCOPy:CWINdow"}, {"Level"=2, "Class Only"=FALSE, "Identifier"="RSRTX_ATTR_HARDCOPY_DEVICE_LANGUAGE_OUTPUT_FORMAT", "Descriptive Name"="Hardcopy Device Language Output Format", "Data Type"=0, "Command"="HCOP:LANG", "Access"=2, "Range Table"="rsrtx_rngHardcopyDeviceLang", "Read Callback"="", "Write Callback"="", "Supported Models"="", "Instrument Options"="", "Flags"=0, "Help"="Defines the file format for the image of the display.\n\nAvailable Repeated Capabilities:\nNone\n\nRemote-control command(s):\nHCOPy:LANGuage"}, {"Level"=2, "Class Only"=FALSE, "Identifier"="RSRTX_ATTR_HARDCOPY_OUTPUT_FORMAT", "Descriptive Name"="Hardcopy Output Format", "Data Type"=0, "Command"="HCOP:FORM", "Access"=2, "Range Table"="rsrtx_rngHardcopyFormat", "Read Callback"="", "Write Callback"="", "Supported Models"="", "Instrument Options"="", "Flags"=0, "Help"="Defines the file format for the image of the display.\n\nAvailable Repeated Capabilities:\nNone\n\nRemote-control command(s):\nHCOPy:FORMat"}, {"Level"=2, "Class Only"=FALSE, "Identifier"="RSRTX_ATTR_HARDCOPY_DEVICE_ORIENTATION", "Descriptive Name"="Hardcopy Device Orientation", "Data Type"=0, "Command"="HCOP:PAGE:ORI", "Access"=2, "Range Table"="rsrtx_rngHardcopyDeviceOrientation", "Read Callback"="", "Write Callback"="", "Supported Models"="", "Instrument Options"="", "Flags"=0, "Help"="Defines the page orientation.\n\nAvailable Repeated Capabilities:\nNone\n\nRemote-control command(s):\nHCOPy:PAGE:ORIentation"}, {"Level"=2, "Class Only"=FALSE, "Identifier"="RSRTX_ATTR_HARDCOPY_PAGE_SIZE_X", "Descriptive Name"="Hardcopy Page Size X", "Data Type"=0, "Command"="HCOP:SIZE:X?", "Access"=0, "Range Table"="", "Read Callback"="", "Write Callback"="", "Supported Models"="", "Instrument Options"="", "Flags"=0, "Help"="Queries X size of the page.\n\nAvailable Repeated Capabilities:\nNone\n\nRemote-control command(s):\nHCOPy:SIZE:X?"}, {"Level"=2, "Class Only"=FALSE, "Identifier"="RSRTX_ATTR_HARDCOPY_PAGE_SIZE_Y", "Descriptive Name"="Hardcopy Page Size Y", "Data Type"=0, "Command"="HCOP:SIZE:Y?", "Access"=0, "Range Table"="", "Read Callback"="", "Write Callback"="", "Supported Models"="", "Instrument Options"="", "Flags"=0, "Help"="Queries Y size of the page.\n\nAvailable Repeated Capabilities:\nNone\n\nRemote-control command(s):\nHCOPy:SIZE:Y?"}, {"Level"=2, "Class Only"=FALSE, "Identifier"="RSRTX_ATTR_HARDCOPY_PRINT", "Descriptive Name"="Hardcopy Print", "Data Type"=4, "Command"="HCOP:IMM", "Access"=1, "Range Table"="", "Read Callback"="", "Write Callback"="", "Supported Models"="", "Instrument Options"="", "Flags"=1, "Help"="Prints an image of the display to the printer or saves an image to a file or the clipboard, depending on the RSRTX_ATTR_HARDCOPY_DEVICE_DESTINATION attribute.\nThe printer 
